vi "Calibration.vi"(0 "Numeric":dbl, 2 "Apply calibration":bool, 3 "SLM colour coding":enum16{"8-bit", "10-bit (Santec)"}(ring)=enum."10-bit (Santec)", 4 "Calibration Path":path=path "C:/GitRepositories/uOttawa/slmcontrol/Untitled.bmp", 5 "Input hologram":u8[][](graph)) -> (1 "Output hologram":dbl[][](graph))   [LabVIEW 2024]
panel:
  out "Coding":dbl
  out "output array 3":i64[][](array[numeric])
  out "Hologram sizes":i32[](array[numeric])
  out "Calibration sizes":i32[](array[numeric])
  out "Output hologram (without modulo)":dbl[][](graph)
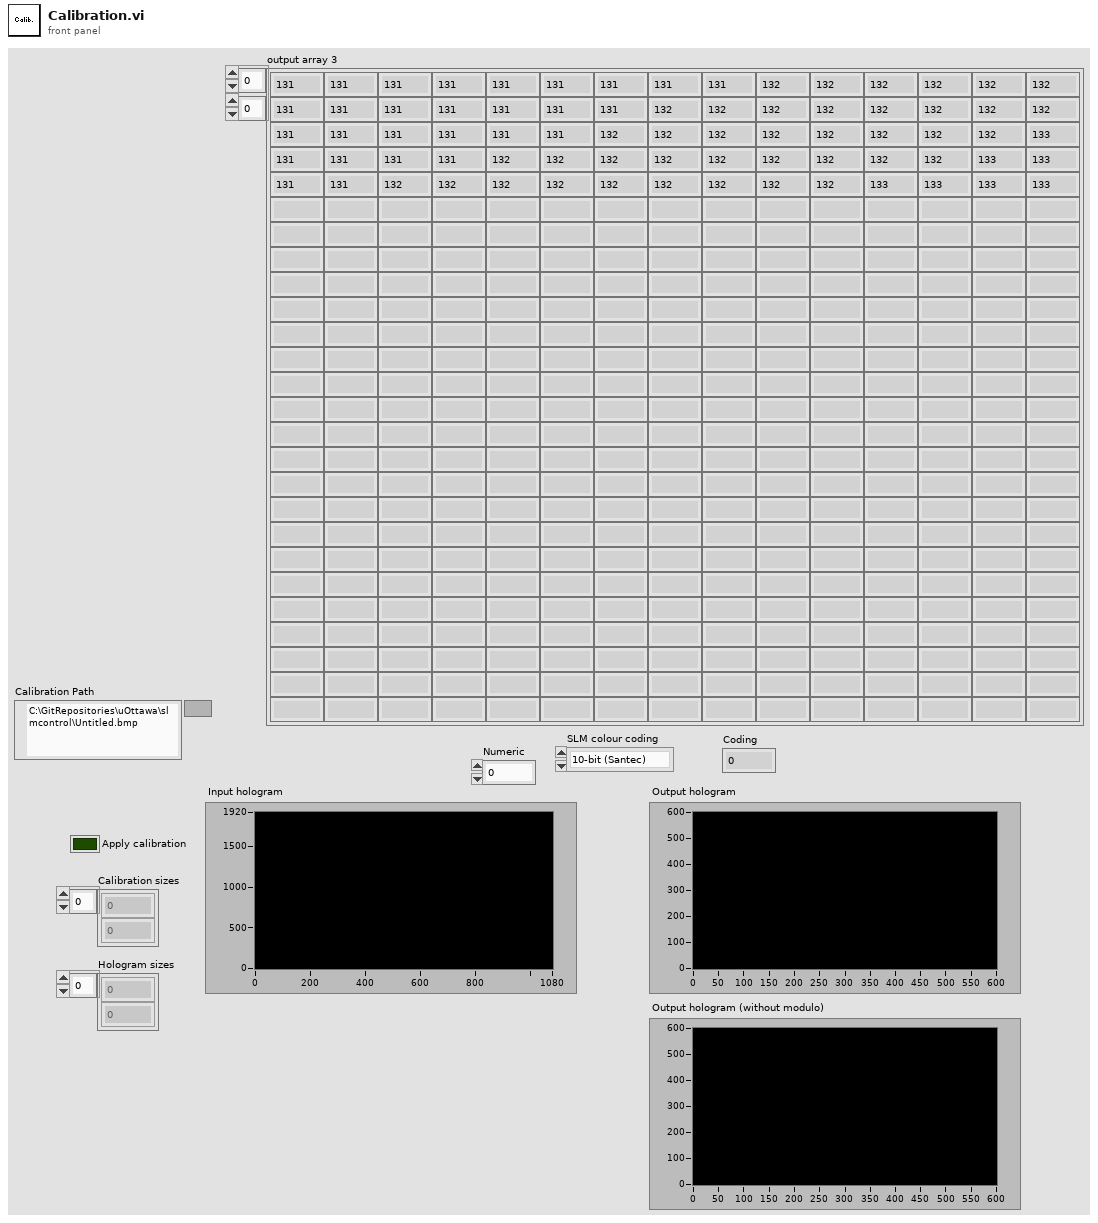
[diagram p1: front panel]
types:
  T1 = typedef "imagedata.ctl" = cluster{"image type":i32, "image depth":i32, "image":u8[], "mask":u8[], "colors":u32[], "Rectangle":cluster{"left":i16, "top":i16, "right":i16, "bottom":i16}}
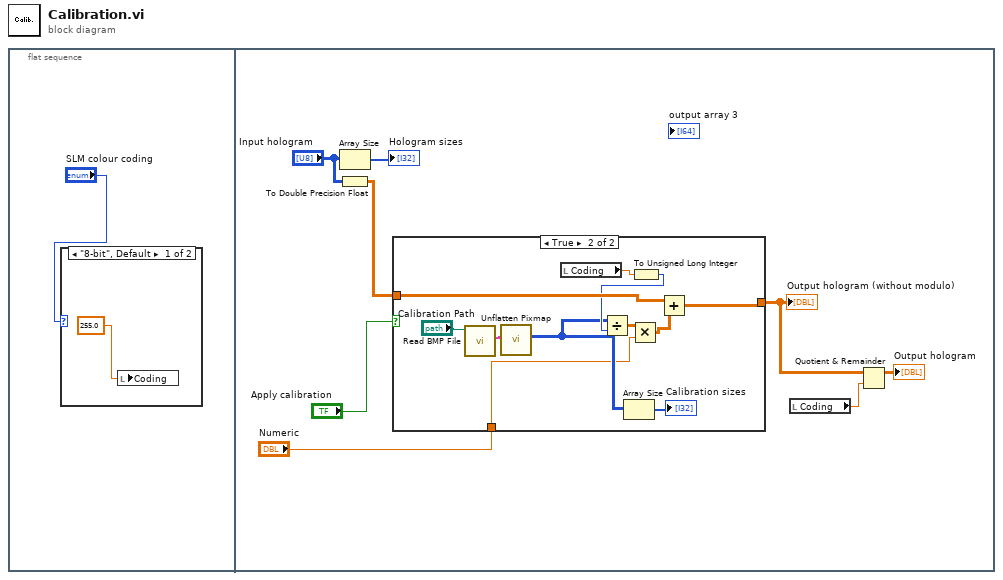
[diagram p0: block diagram]
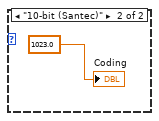
[diagram p2: hidden frame]
diagram:
  n1 = flat-sequence {
    frame #0 {
      n2 = case shown="\"8-bit\", Default" "SLM colour coding" {
        frame "8-bit", Default {
          n3 = local write "Coding"(255.0) -> ()
        }
        frame "10-bit (Santec)" {
          "Coding" <- 1023.0
        }
      }
    }
    frame #1 {
      n4 = Array Size(array="Input hologram") -> (size(s)=→"Hologram sizes":i32[])
      n5 = To Double Precision Float(number="Input hologram") -> (double precision float=w10:dbl[][])
      n6 = case shown="True" "Apply calibration" {
        tunnel: w10 -> [w12 w23]
        tunnel: [w12 w22] -> w9
        tunnel: "Numeric" -> [_ w13]
        frame False {
        }
        frame True {
          n7 = call <vilib>:"Read BMP File.vi"("path to BMP file"="Calibration Path") -> ("image data"=w15:T1)  [unwired: 8 in, 2 out]
          n8 = call <vilib>:"Unflatten Pixmap.vi"("image data"=w15) -> ("8-bit pixmap"=w14:u8[][])  [unwired: 4 in, 6 out]
          n9 = local read "Coding"() -> (w19:dbl)
          n10 = Array Size(array=w14) -> (size(s)=→"Calibration sizes":i32[])
          n11 = To Unsigned Long Integer(number=w19) -> (unsigned 32bit integer=w18:u32)
          n12 = Divide(x=w14, y=w18) -> (x/y=w20:dbl[][])
          n13 = Multiply(x=w20, y=w13) -> (x*y=w21:dbl[][])
          n14 = Add(x=w23, y=w21) -> (x+y=w22:dbl[][])
        }
      }
      "Output hologram (without modulo)" <- w9
      n15 = local read "Coding"() -> (w6:dbl)
      n16 = Quotient & Remainder(x=w9, y=w6) -> (x-y*floor(x/y)=→"Output hologram":dbl[][])  [unwired: 1 out]
    }
  }
